vi "WS1050 OFFSET CAL.vi"(8 "error in":errorcluster, 10 "OFFSET CAL":bool=TRUE) -> (0 "error out":errorcluster, 3 "AD7747 Values":string[][](table))   [LabVIEW 2012]
uses:
  Type Defs/WSVCAP SHL I2C DUT Mask Mode Enum.ctl
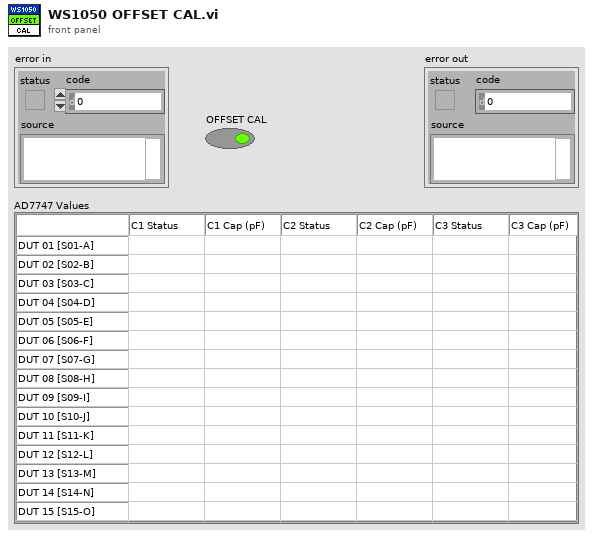
[diagram p1: front panel]
types:
  T1 = typedef "WSVCAP SHL I2C DUT Mask Mode Enum.ctl" = enum16{"Custom", "C1", "C2", "C3", "All"}
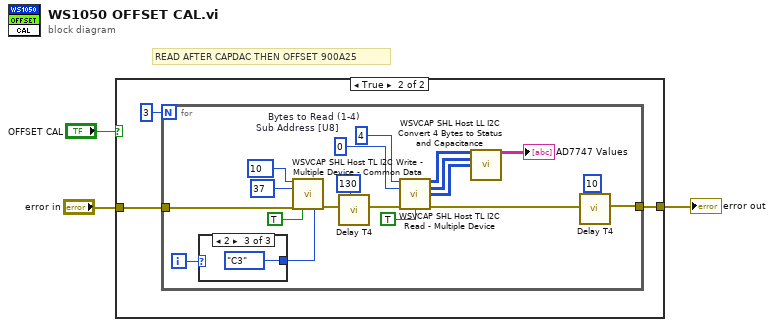
[diagram p0: block diagram]
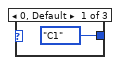
[diagram p3: hidden frame]
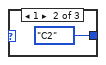
[diagram p4: hidden frame]
diagram:
  # "READ AFTER CAPDAC THEN OFFSET 900A25"
  n1 = case shown="True" "OFFSET CAL" {
    tunnel: "error in" -> [w4 w7]
    tunnel: [w4 w6] -> w3
    frame False {
    }
    frame True {
      n2 = for {
        N: 3 -> [_]
        tunnel: w7 -> [w26]
        tunnel: [w12] -> w6
        i -> [w9]
        w24 = u8 4  # Bytes to Read (1-4)
        w25 = u8 0  # Sub Address [U8]
        n3 = case shown="2" w9 {
          tunnel: [WSVCAP_SHL_I2C_DUT_Mask_Mode_Enum."C1" ("DUT Mask Mode (All)") WSVCAP_SHL_I2C_DUT_Mask_Mode_Enum."C2" ("DUT Mask Mode (All)") WSVCAP_SHL_I2C_DUT_Mask_Mode_Enum."C3" ("DUT Mask Mode (All)")] -> w8
          frame 0, Default {
          }
          frame 1 {
          }
          frame 2 {
          }
        }
        n4 = call "WSVCAP SHL Host TL I2C Write - Multiple Device - Common Data.vi"("Sub Address"=u8 10, "Data Out [U8]"=u8 37 ("Sub Address"), "error in"=w26, "Log (T)"=TRUE, "DUT Mask Mode (All)"=w8) -> ("error out"=w14:errorcluster)  [unwired: 10 in]
        n5 = call "Delay T4.vi"("milliseconds to wait"=u32 130, "error in (no error)"=w14) -> ("error out"=w15:errorcluster)  [unwired: 9 in]
        n6 = call "WSVCAP SHL Host TL I2C Read - Multiple Device.vi"("Bytes to Read (1-4)"=w24, "Sub Address [U8]"=w25, "error in"=w15, "Log (T)"=TRUE) -> ("C1:1-16 Read Data [U8]"=w23:u8[][], "C2:1-16 Read Data [U8]"=w22:u8[][], "C3:1-16 Read Data [U8]"=w20:u8[][], "error out"=w11:errorcluster)  [unwired: 8 in]
        n7 = call "WSVCAP SHL Host LL I2C Convert 4 Bytes to Status and Capacitance.vi"("C1:1-16 Read Data [U8]"=w23, "C2_1-16 Read Data [U8]"=w22, "C3_1-16 Read Data [U8]"=w20) -> ("AD7747 Values"=→"AD7747 Values":string[][])  [unwired: 12 in]
        n8 = call "Delay T4.vi"("milliseconds to wait"=u32 10, "error in (no error)"=w11) -> ("error out"=w12:errorcluster)  [unwired: 9 in]
      }
    }
  }
  "error out" <- w3
